vi "Get_Recipes.vi"(8 "error in (no error)":errorcluster) -> (0 "error out":errorcluster, 3 "Recipes":string[][](array[string]))   [LabVIEW 2026]
doc: "The Get_Recipes.vi reads the recipes.csv from the home directory, placing the details (name, time, and power levels) into a 2D-string array."
uses:
  <vilib>/Utility/file.llb/Read Delimited Spreadsheet (string).vi
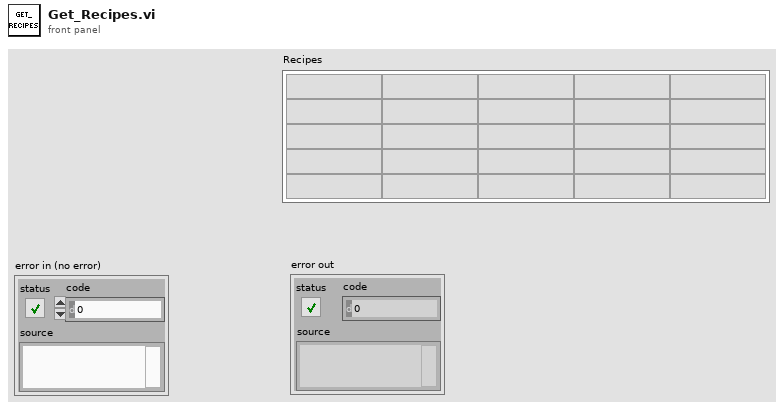
[diagram p1: front panel]
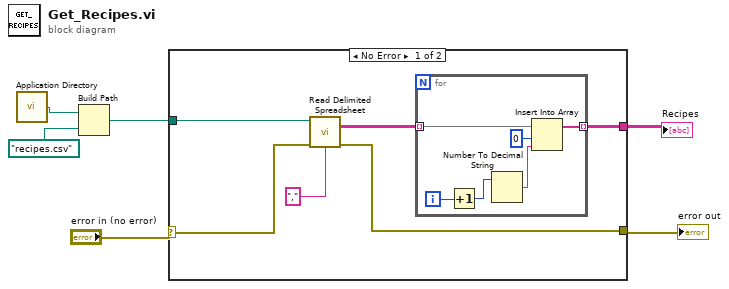
[diagram p0: block diagram]
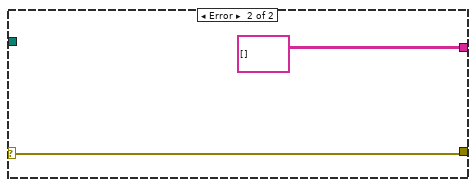
[diagram p2: hidden frame]
diagram:
  n1 = call <vilib>:"Application Directory.vi"() -> ("Application Directory"=w6:path)
  n2 = Build Path(base path=w6, name or relative path=path "recipes.csv") -> (appended path=w3:path)
  n3 = case shown="No Error" "error in (no error)" {
    selector: "error in (no error)" -> [w10 w19]
    tunnel: w3 -> [w12 _]
    tunnel: [w7 string[][] [] ("all rows")] -> w2
    tunnel: [w9 w19] -> w1
    frame No Error {
      n4 = call-poly <vilib>:"Read Delimited Spreadsheet.vi"("file path (dialog if empty)"=w12, "error in (no error)"=w10, "delimiter (\\t)"="," ("delimiter (\\t)")) -> ("all rows"=w8:string[][], "error out"=w9:errorcluster)  [unwired: 7 in, 4 out]
      n5 = for {
        tunnel: w8 -> [w18] mode=indexing
        tunnel: [w15] -> w7 mode=indexing
        i -> [w14]
        n6 = Increment(x=w14) -> (x+1=w17:i32)
        n7 = Number To Decimal String(number=w17) -> (decimal integer string=w16:string)  [unwired: 1 in]
        n8 = Insert Into Array(array=w18, index=0, new element=w16) -> (w15:string[])
      }
    }
    frame Error {
    }
  }
  "Recipes" <- w2
  "error out" <- w1
